vi "Read Sample name.vi"(8 "error in (no error)":errorcluster, 11 "Data3D in":refnum<class "Data3D.lvclass">) -> (0 "error out":errorcluster, 2 "Sample name":string, 3 "Data3D out":refnum<class "Data3D.lvclass">)   [LabVIEW 2014, in "Data3D.lvclass"]
uses:
  Data3D.lvclass
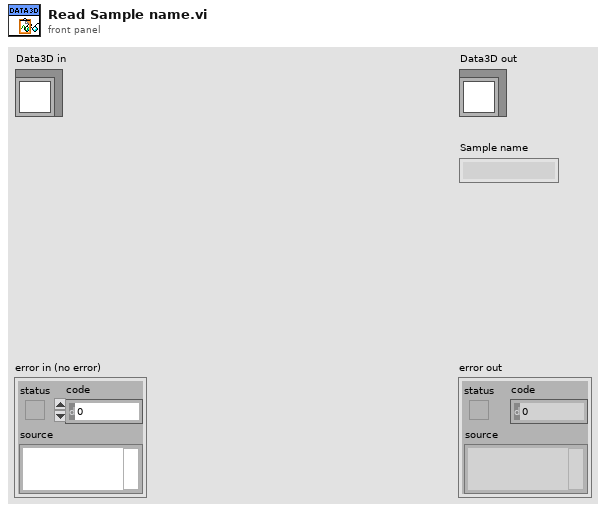
[diagram p1: front panel]
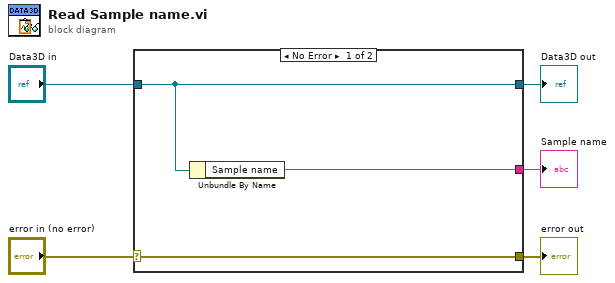
[diagram p0: block diagram]
diagram:
  n1 = case shown="No Error" "error in (no error)" {
    selector: "error in (no error)" -> [w8 w9]
    tunnel: [w8 w9] -> w4
    tunnel: [w7 w10] -> w2
    tunnel: "Data3D in" -> [w7 w10]
    tunnel: [w6 _] -> w1
    frame No Error {
      n2 = Unbundle By Name(w7) -> ("Sample name"=w6:string)
    }
    frame Error {
    }
  }
  "error out" <- w4
  "Data3D out" <- w2
  "Sample name" <- w1
